vi "Canbus frame cluster to LEIN.vi"(7 "CAN FRAME TIMED":T1 {"Data" format="%.0x"; "ArbitrationId" format="%.0x"; "Timestamp" format="%<%I:%M:%S%3u %p\n%m/%d/%Y>T"}, 11 "error in (no error)":errorcluster) -> (8 "CMD":T2={"SID"=0, "ANF"=FALSE, "CMD"=enum."TASK", "DATA"=[]}, 10 "LEIN Frame":bool, 15 "error out":errorcluster)   [LabVIEW 2010]
uses:
  Defenitions/LEIN CMD Cluster.ctl
  Defenitions/LEIN CMD List.ctl
  <vilib>/nican/nican.llb/CanFrameTimed.ctl
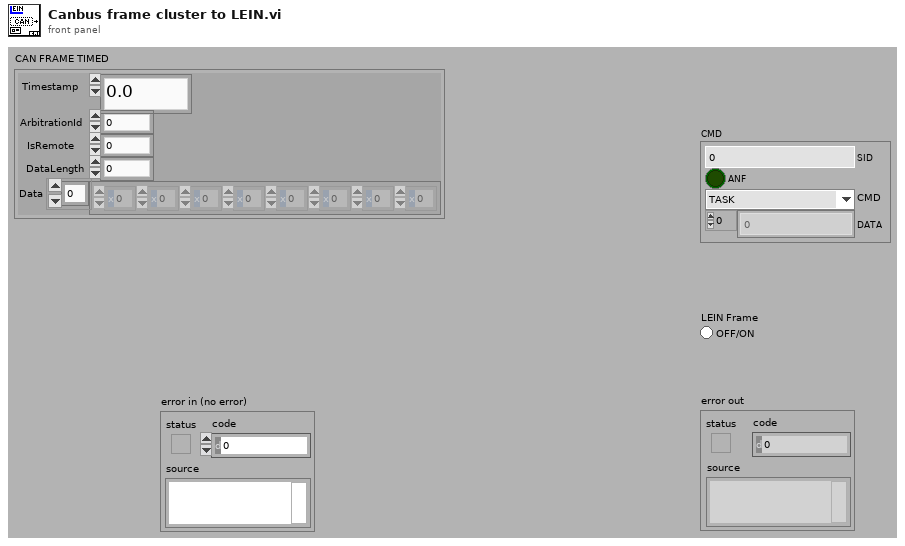
[diagram p1: front panel]
types:
  T1 = typedef "CanFrameTimed.ctl" = cluster{"Timestamp":dbl, "ArbitrationId":u32, "IsRemote":u8, "DataLength":u8, "Data":u8[]}
  T2 = typedef "LEIN CMD Cluster.ctl" = cluster{"SID":u8, "ANF":bool, "CMD":T3, "DATA":u8[]}
  T3 = typedef "LEIN CMD List.ctl" = enum8{"ACTI", "TASK", "RES0", "STAT", "RES1", "RES2", "RES3", "USER"}
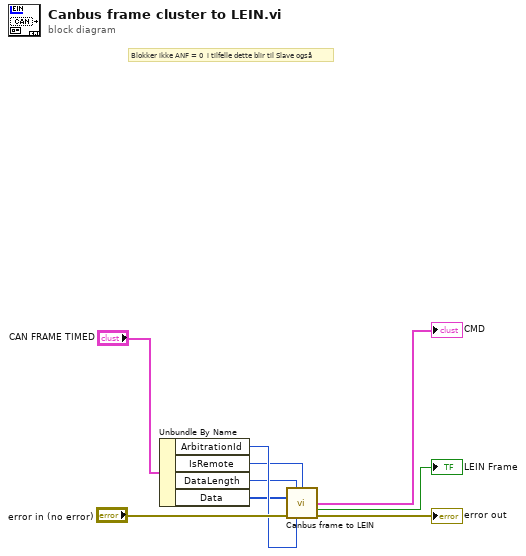
[diagram p0: block diagram]
diagram:
  # "Blokker ikke ANF = 0  i tilfelle dette blir til Slave også"
  n1 = Unbundle By Name("CAN FRAME TIMED") -> ("ArbitrationId"=w7:u32, "IsRemote"=w6:u8, "DataLength"=w5:u8, "Data"=w4:u8[])
  n2 = call "Canbus frame to LEIN.vi"("Data Length"=w5, "IsRemote(0)"=w6, "Data"=w4, "error in (no error)"="error in (no error)", "ArbitrationID"=w7) -> ("CMD"=→"CMD":T2, "LEIN Frame"=→"LEIN Frame":bool, "error out"=→"error out":errorcluster)  [unwired: 8 in]
